vi "Capacitance PID-LS340.vi"() -> ()   [LabVIEW 2020]
doc: "This VI is meant to be used with the process control package (PID controller) and an MIO-series or Lab-PC data acquisition board. Connect the analog output to the analog input through the resistor-capacitor network shown on the front panel (scroll down to view it). The VI attempts to adjust the analog output so that the input (process variable or PV) equals the setpoint (SP). SP and PV are displayed on a strip chart. You can experiment with different controller tuning methods and try for the fastest settling time with the least overshoot.\n\nThe input span is -10 to +10 V, or 20V = 100%. The output span is 0 to +10 V, or 10V = 100%. PV and SP are in Volts. Your MIO board should be set up for differential input and -10 to +10 V range; the output should be unipolar, 10V (these are all factory defaults). If you elect to use other settings, run the configuration VIs as necessary.\n\nThe recommended network has a DC gain of 0.33, an effective deadtime of about 5 Sec., and an effective time constant of about 30 Sec."
uses:
  <vilib>/addons/control/pid/NI_PID__autopid compat.lvlib
panel:
  out "Trend 2":dbl(graph)=18.537378083708255
  in  "Heater Range":i32(ring)=2 items=["Off", "31.6 uA", "100 uA", "316 uA", "1.00 mA", "3.16 mA", "10.0 mA", "31.6 mA", "100 mA"]
  in  "Lakeshore GPIB Address":refnum<visa-resource-name>="GPIB0::5::INSTR"
  out "Cycle #":i32=301
  in  "Bias":dbl format="%.2f"
  in  "gain scheduling":T1={"gain schedule"=[1.0], "PID parameters"=[{"Kc"=3.0, "Ti (min)"=0.5, "Td (min)"=0.0}], "scheduling input"=0} {"scheduling input" items=["Setpoint", "Process variable", "Controller output", "Gain scheduling input"]; "PID parameters"."Td (min)" format="%.4f"; "PID parameters"."Ti (min)" format="%.4f"; "PID parameters"."Kc" format="%#.3f"; "gain schedule" format="%.2f"}
  in  "?":bool
  in  "options":T2={"sp low"=1600.0, "sp high"=1800.0, "out low"=0.0, "out high"=100.0, "hold (F)"=FALSE, "auto (T)"=TRUE, "pro. band (F)"=FALSE, "reverse acting (T)"=TRUE, "beta"=1.0, "linearity"=1.0, "dt (s)"=-1.0} {"dt (s)" format="%.2f"; "linearity" min=0.0 max=1.0 format="%.2f"; "sp low" format="%.2f"; "sp high" format="%.2f"; "out low" format="%.2e"; "out high" format="%.2e"; "beta" min=0.0 max=1.0 format="%.2f"}
  in  "STOP":bool
  in  "Setpoint (pF)":dbl(slide)=1764.0 min=1600.0 max=1800.0 step=0.0001 scale=1600.0..1800.0 scale format="%.2f"
  out "Output (W)":dbl(slide)=18.537378083708255 scale=0.0..100.0 scale format="%#.2p"
  in  "Cycle Time (sec)":dbl=3.0 format="%.2f"
  in  "Manual Out (W)":dbl(knob)=18.537378083708255 min=-4e-06 max=4e-06 scale=-100.0..100.0 scale format="%#.2p"
  out "Trend":cluster{"Setpoint (V)":dbl, "Setpoint (V)":dbl}(graph)={"Setpoint (V)"=1763.9007, "Setpoint (V)"=1764.0}
  # "SP & PV range:"
  # "Output range:"
  # "-1: default,using\nsystem clock"
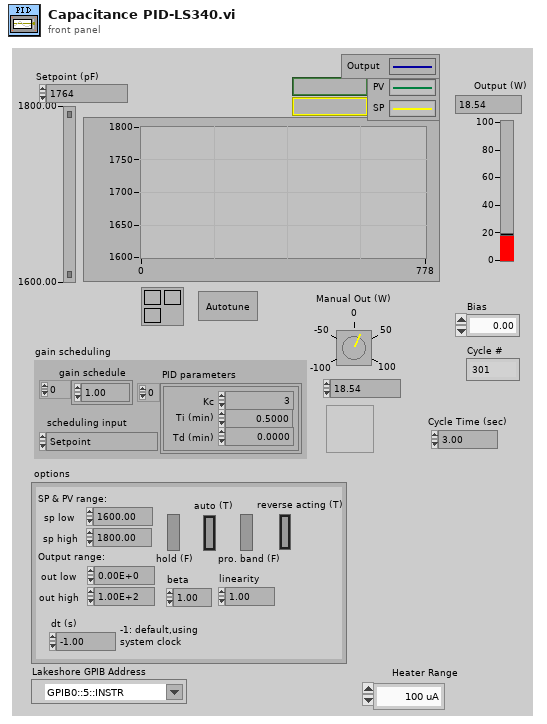
[diagram p1: front panel]
types:
  T1 = cluster{"gain schedule":dbl[], "PID parameters":cluster{"Kc":dbl, "Ti (min)":dbl, "Td (min)":dbl}[], "scheduling input":u16}
  T2 = cluster{"sp low":dbl, "sp high":dbl, "out low":dbl, "out high":dbl, "hold (F)":bool, "auto (T)":bool, "pro. band (F)":bool, "reverse acting (T)":bool, "beta":dbl, "linearity":dbl, "dt (s)":dbl}
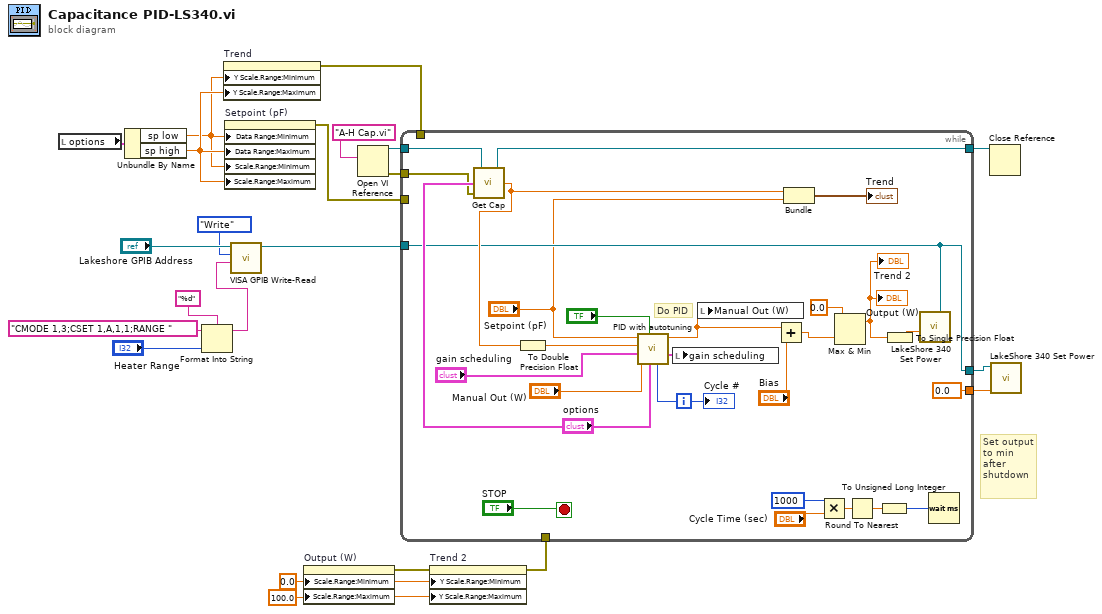
[diagram p0: block diagram]
diagram:
  w1 = 100.0 ("Scale.Range:Maximum")
  w5 = 0.0 ("Scale.Range:Minimum")
  # "Set output \nto min after shutdown"
  n1 = local read "options"() -> (w9:T2)
  n2 = Unbundle By Name(w9) -> ("sp low"=w3:dbl, "sp high"=w4:dbl)
  n3 = Format Into String(format string="%d" ("initial string"), initial string="CMODE 1,3;CSET 1,A,1,1;RANGE ", "Heater Range") -> (resulting string=w12:string)  [unwired: 1 in, 1 out]
  n4 = property on="Trend" class="WFChart (strict)"("Y Scale.Range:Minimum"=w3, "Y Scale.Range:Maximum"=w4) -> (error out=w2:errorcluster)  [unwired: 2 in, 1 out]
  n5 = property on="Setpoint (pF)" class="Slide (strict)"("Data Range:Minimum"=w3, "Data Range:Maximum"=w4, "Scale.Range:Minimum"=w3, "Scale.Range:Maximum"=w4) -> (error out=w8:errorcluster)  [unwired: 2 in, 1 out]
  n6 = call "VISA GPIB Write-Read.vi"("Command"=w12, "Action"=enum16{"Write", "Read", "Write & Read"}."Write", "VISA resource name"="Lakeshore GPIB Address") -> ("dup VISA Session"=w15:refnum<visa-resource-name>)  [unwired: 5 in, 3 out]
  n7 = property on="Output (W)" class="Slide (strict)"("Scale.Range:Minimum"=w5, "Scale.Range:Maximum"=w1) -> (error out=w7:errorcluster)  [unwired: 2 in, 1 out]
  n8 = Open VI Reference(vi path="A-H Cap.vi") -> (vi reference=w19:refnum<vi>, error out=w17:errorcluster)  [unwired: 5 in]
  n9 = property on="Trend 2" class="WFChart (strict)"(error in=w7, "Y Scale.Range:Minimum"=w5, "Y Scale.Range:Maximum"=w1) -> (error out=w6:errorcluster)  [unwired: 1 in, 1 out]
  n10 = while {
    tunnel: w17 -> [w35]
    tunnel: [w37] -> w18
    tunnel: w19 -> [w38]
    tunnel: [sgl 0.0] -> w21
    tunnel: [w28] -> w22
    tunnel: w15 -> [w28]
    tunnel: w8 -> [_]
    tunnel: w6 -> [_]
    tunnel: w2 -> [_]
    i -> [w43]
    stop <- "STOP" stop-if-true
    # "Do PID"
    n11 = call "Get Cap.vi"("error in"=w35, "options"="options", "VI Refnum 2"=w38) -> ("Setpoint (V)"=w34:dbl, "VI Refnum"=w37:refnum<vi>)  [unwired: 1 in]
    n12 = To Double Precision Float(number=w34) -> (double precision float=w39:dbl)
    n13 = call <vilib>:"PID with autotuning.vi"("iteration"=w43, "options"="options", "autotune? (F)"="?", "manual control"="Manual Out (W)", "gain scheduling"="gain scheduling", "process variable"=w39, "setpoint"="Setpoint (pF)") -> ("updated parameters"=w42:T1, "output"=w32:dbl)  [unwired: 2 in, 1 out]
    n14 = local write "gain scheduling"(w42) -> ()
    n15 = local write "Manual Out (W)"(w32) -> ()
    n16 = Add(x=w32, y="Bias") -> (x+y=w23:dbl)
    n17 = Bundle("Setpoint (V)"=w34, "Setpoint (pF)"="Setpoint (pF)") -> (→"Trend":cluster{"Setpoint (V)":dbl, "Setpoint (pF)":dbl})  [unwired: 1 in]
    n18 = Multiply(x=1000, y="Cycle Time (sec)") -> (x*y=w46:dbl)
    n19 = Max & Min(x=0.0, y=w23) -> (max(x,y)=w25:dbl)  [unwired: 1 out]
    "Output (W)" <- w25
    "Trend 2" <- w25
    n20 = Round To Nearest(number=w46) -> (nearest integer value=w31:dbl)
    n21 = To Unsigned Long Integer(number=w31) -> (unsigned 32bit integer=w30:u32)
    n22 = To Single Precision Float(number=w25) -> (single precision float=w26:sgl)
    n23 = call "LakeShore 340 Set Power.vi"("Heater Power (W)"=w26, "Lakeshore GPIB Address"=w28) -> ()  [unwired: 3 in, 1 out]
    n24 = Wait (ms)(milliseconds to wait=w30) -> ()  [unwired: 1 out]
    "Cycle #" <- w43
  }
  n25 = Close Reference(reference=w18) -> ()  [unwired: 1 in, 1 out]
  n26 = call "LakeShore 340 Set Power.vi"("Heater Power (W)"=w21, "Lakeshore GPIB Address"=w22) -> ()  [unwired: 3 in, 1 out]
